vi "AnalogInput-Array.vi"() -> ()   [LabVIEW 2017]
uses:
  <vilib>/DAQmx/read.llb/DAQmx Read (Analog 1D DBL 1Chan NSamp).vi
  <vilib>/DAQmx/create/channels.llb/DAQmx Create Channel (AI-Voltage-Basic).vi
  <vilib>/DAQmx/configure/timing.llb/DAQmx Timing (Sample Clock).vi
  <vilib>/DAQmx/miscellaneous.llb/DAQmx Fill In Error Info.vi
panel:
  out "Loop Time in ms":u32
  in  "Boolean":bool
  in  "number of samples per channel":i32=2000
  out "Waveform Graph":dbl[](graph)
  out "error out":errorcluster
  in  "rate":dbl=1000.0 format="%0.2f"
  in  "physical channels":tag
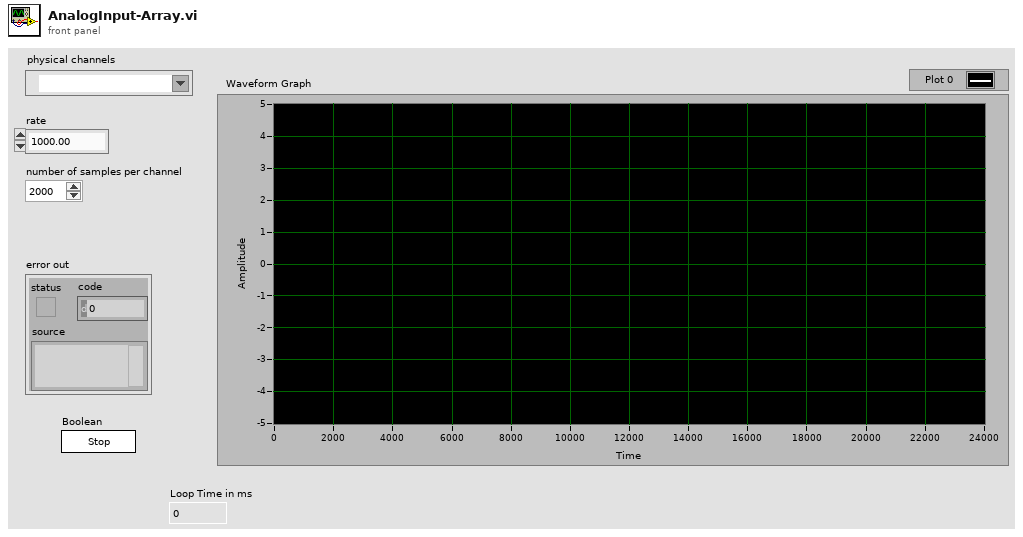
[diagram p1: front panel]
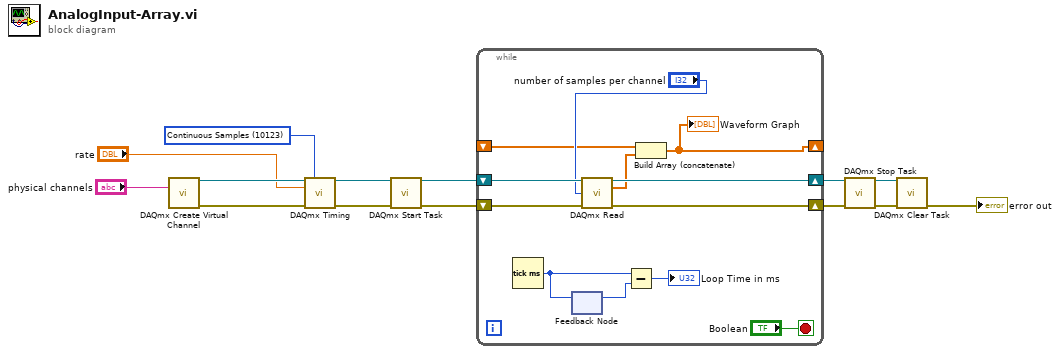
[diagram p0: block diagram]
diagram:
  w10 = 10123 items=["Finite Samples"=10178, "Continuous Samples"=10123, "Hardware Timed Single Point"=12522] ("sample mode")
  n1 = call-poly <vilib>:"DAQmx Create Virtual Channel.vi"("physical channels"="physical channels") -> ("task out"=w13:refnum<k21>, "error out"=w12:errorcluster)  [unwired: 13 in]
  n2 = call-poly <vilib>:"DAQmx Timing.vi"("task/channels in"=w13, "sample mode"=w10, "rate"="rate", "error in"=w12) -> ("task out"=w2:refnum<k21>, "error out"=w9:errorcluster)  [unwired: 10 in]
  n3 = call <vilib>:"DAQmx Start Task.vi"("task/channels in"=w2, "error in"=w9) -> ("task out"=w1:refnum<k21>, "error out"=w3:errorcluster)  [unwired: 12 in]
  n4 = while {
    shift-right: [w24] -> w5
    shift-left: w1 -> [w26]
    shift-right: [w23] -> w8
    shift-left: w3 -> [w25]
    shift-right: [w15] -> _
    shift-left: _ -> [w16]
    stop <- "Boolean" stop-if-true
    n5 = Tick Count (ms)() -> (millisecond timer value=w21:u32)
    n6 = feedback-in #1(w21) -> ()
    n7 = feedback #1() -> (w20:u32)  [unwired: 1 in]
    n8 = call-poly <vilib>:"DAQmx Read.vi"("task/channels in"=w26, "number of samples per channel"="number of samples per channel", "error in"=w25) -> ("task out"=w24:refnum<k21>, "data"=w18:dbl[], "error out"=w23:errorcluster)  [unwired: 10 in]
    n9 = Subtract(x=w21, y=w20) -> (x-y=→"Loop Time in ms":u32)
    n10 = Build Array (concatenate)(w16, w18) -> (w15:dbl[])
    "Waveform Graph" <- w15
  }
  n11 = call <vilib>:"DAQmx Stop Task.vi"("task/channels in"=w5, "error in"=w8) -> ("task out"=w4:refnum<k21>, "error out"=w6:errorcluster)  [unwired: 12 in]
  n12 = call <vilib>:"DAQmx Clear Task.vi"("task in"=w4, "error in"=w6) -> ("error out"=→"error out":errorcluster)  [unwired: 13 in]
